vi "Wire N Reserve Session Inputs.vi"(0 "sub vi in":refnum<vi>, 5 "vi reference":refnum<vi>, 7 "build array":refnum<vi>, 11 "error in":errorcluster) -> (15 "error out":errorcluster)   [LabVIEW 2021, in "Converter.lvlib"]
uses:
  Converter.lvlib
  Converter Reusables/Converter Reusables.lvlib
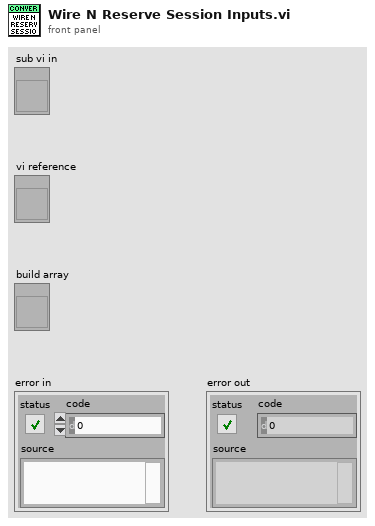
[diagram p1: front panel]
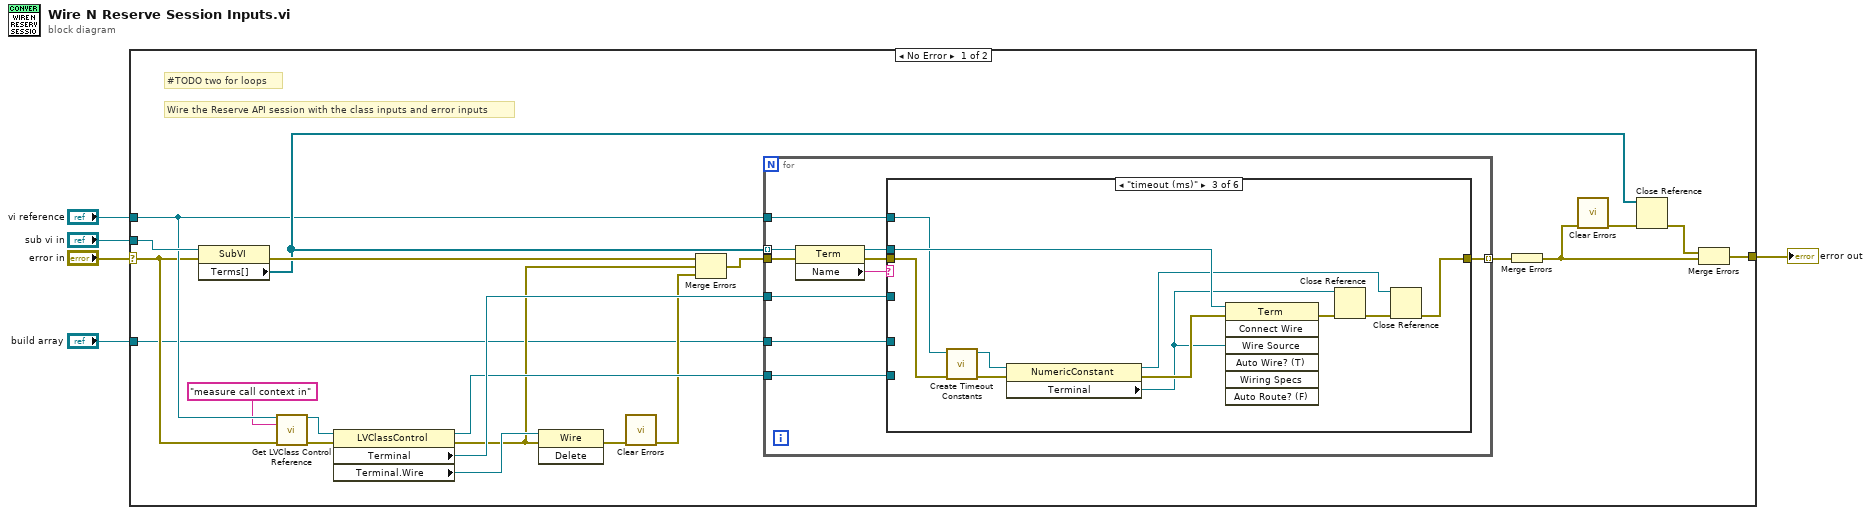
[diagram p0: block diagram]
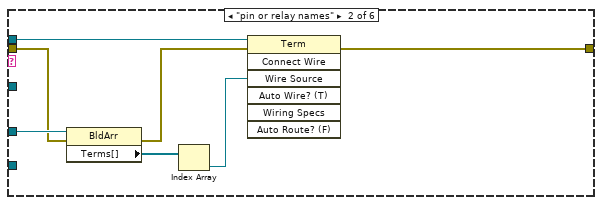
[diagram p3: hidden frame]
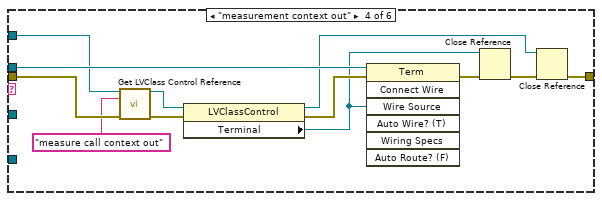
[diagram p4: hidden frame]
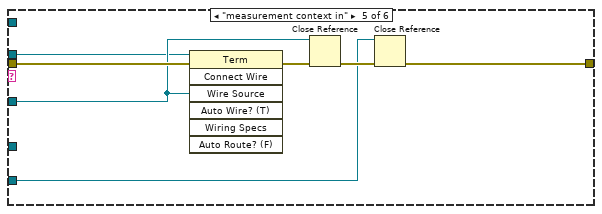
[diagram p5: hidden frame]
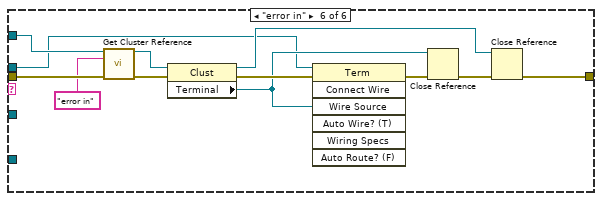
[diagram p6: hidden frame]
diagram:
  n1 = case shown="No Error" "error in" {
    selector: "error in" -> [w12 w87]
    tunnel: "sub vi in" -> [w24 _]
    tunnel: [w20 w87] -> w1
    tunnel: "vi reference" -> [w16 _]
    tunnel: "build array" -> [w6 _]
    frame No Error {
      # "Wire the Reserve API session with the class inputs and error inputs"
      # "#TODO two for loops"
      n2 = property class="SubVI"(reference=w24, error in=w12) -> (error out=w25:errorcluster, "Terms[]"=w23:refnum<vi>[])  [unwired: 1 out]
      n3 = call "Get LVClass Control Reference.vi"("vi in"=w16, "name/order"="measure call context in", "error in"=w12) -> ("cluster out"=w14:refnum<vi>, "error out"=w17:errorcluster)  [unwired: 11 in]
      n4 = property class="LVClassControl"(reference=w14, error in=w17) -> (reference out=w13:refnum<vi>, error out=w10:errorcluster, "Terminal"=w15:refnum<vi>, "Terminal.Wire"=w18:refnum<vi>)
      n5 = invoke class="Wire" method="Delete"(reference=w18, error in=w10) -> (error out=w9:errorcluster)  [unwired: 1 in, 2 out]
      n6 = call <vilib>:"Clear Errors.vi"("error in (no error)"=w9) -> ("error out"=w8:errorcluster)  [unwired: 5 in, 1 out]
      n7 = Merge Errors(w25, w10, w8) -> (w11:errorcluster)
      n8 = for {
        tunnel: w23 -> [w36] mode=indexing
        tunnel: w11 -> [w35]
        tunnel: [w31] -> w26 mode=indexing
        tunnel: w16 -> [w30]
        tunnel: w6 -> [w29]
        tunnel: w15 -> [w28]
        tunnel: w13 -> [w27]
        n9 = property class="Term"(reference=w36, error in=w35) -> (reference out=w32:refnum<vi>, error out=w33:errorcluster, "Name"=w34:string)
        n10 = case shown="\"timeout (ms)\"" w34 {
          tunnel: w33 -> [w37 w40 w46 w64 w74 w85]
          tunnel: w32 -> [_ w44 w55 w67 w68 w75]
          tunnel: [w37 w43 w52 w60 w71 w82] -> w31
          tunnel: w30 -> [_ _ w51 w59 _ w76]
          tunnel: w29 -> [_ w41 _ _ _ _]
          tunnel: w28 -> [_ _ _ _ w69 _]
          tunnel: w27 -> [_ _ _ _ w70 _]
          frame Default {
          }
          frame "pin or relay names" {
            n11 = property class="BldArr"(reference=w41, error in=w40) -> (error out=w39:errorcluster, "Terms[]"=w42:refnum<vi>[])  [unwired: 1 out]
            n12 = Index Array(array=w42) -> (element=w38:refnum<vi>)  [unwired: 1 in]
            n13 = invoke class="Term" method="Connect Wire"(reference=w44, error in=w39, "Wire Source"=w38) -> (error out=w43:errorcluster)  [unwired: 4 in, 6 out]
          }
          frame "timeout (ms)" {
            n14 = call "Create Timeout Constants.vi"("error in"=w46, "vi in"=w51) -> ("error out"=w50:errorcluster, "numeric constant out"=w45:refnum<vi>)  [unwired: 8 in]
            n15 = property class="NumericConstant"(reference=w45, error in=w50) -> (reference out=w47:refnum<vi>, error out=w49:errorcluster, "Terminal"=w48:refnum<vi>)
            n16 = invoke class="Term" method="Connect Wire"(reference=w55, error in=w49, "Wire Source"=w48) -> (error out=w54:errorcluster)  [unwired: 4 in, 6 out]
            n17 = Close Reference(reference=w48, error in (no error)=w54) -> (error out=w53:errorcluster)
            n18 = Close Reference(reference=w47, error in (no error)=w53) -> (error out=w52:errorcluster)
          }
          frame "measurement context out" {
            n19 = call "Get LVClass Control Reference.vi"("vi in"=w59, "name/order"="measure call context out", "error in"=w64) -> ("cluster out"=w61:refnum<vi>, "error out"=w65:errorcluster)  [unwired: 11 in]
            n20 = property class="LVClassControl"(reference=w61, error in=w65) -> (reference out=w58:refnum<vi>, error out=w63:errorcluster, "Terminal"=w57:refnum<vi>)
            n21 = invoke class="Term" method="Connect Wire"(reference=w67, error in=w63, "Wire Source"=w57) -> (error out=w66:errorcluster)  [unwired: 4 in, 6 out]
            n22 = Close Reference(reference=w57, error in (no error)=w66) -> (error out=w62:errorcluster)
            n23 = Close Reference(reference=w58, error in (no error)=w62) -> (error out=w60:errorcluster)
          }
          frame "measurement context in" {
            n24 = invoke class="Term" method="Connect Wire"(reference=w68, error in=w74, "Wire Source"=w69) -> (error out=w73:errorcluster)  [unwired: 4 in, 6 out]
            n25 = Close Reference(reference=w69, error in (no error)=w73) -> (error out=w72:errorcluster)
            n26 = Close Reference(reference=w70, error in (no error)=w72) -> (error out=w71:errorcluster)
          }
          frame "error in" {
            n27 = call "Get Cluster Reference.vi"("vi in"=w76, "name/order"="error in", "error in"=w85) -> ("cluster out"=w86:refnum<vi>, "error out"=w84:errorcluster)  [unwired: 11 in]
            n28 = property class="Clust"(reference=w86, error in=w84) -> (reference out=w79:refnum<vi>, error out=w83:errorcluster, "Terminal"=w78:refnum<vi>)
            n29 = invoke class="Term" method="Connect Wire"(reference=w75, error in=w83, "Wire Source"=w78) -> (error out=w80:errorcluster)  [unwired: 4 in, 6 out]
            n30 = Close Reference(reference=w78, error in (no error)=w80) -> (error out=w81:errorcluster)
            n31 = Close Reference(reference=w79, error in (no error)=w81) -> (error out=w82:errorcluster)
          }
        }
      }
      n32 = Merge Errors(w26) -> (w21:errorcluster)
      n33 = call <vilib>:"Clear Errors.vi"("error in (no error)"=w21) -> ("error out"=w19:errorcluster)  [unwired: 5 in, 1 out]
      n34 = Close Reference(reference=w23, error in (no error)=w19) -> (error out=w22:errorcluster)
      n35 = Merge Errors(w22, w21) -> (w20:errorcluster)
    }
    frame Error {
    }
  }
  "error out" <- w1
